vi "Untitled 13 (SubVI).vi"(4 "Порядок фильтра":i64, 5 "Array":dbl[](array[numeric]), 6 "Нижняя частота среза":dbl, 7 "Кол-во выборок":i32, 9 "Переменная floor(x/y)":i32, 10 "Кол-во копий":i32, 11 "Размер окна с паузами":i32) -> (3 "Filtered X":dbl[](array[numeric]))   [LabVIEW 2017]
uses:
  <vilib>/Analysis/3filter.llb/Bessel Filter (DBL).vi
  <vilib>/Analysis/NI_AALBase.lvlib
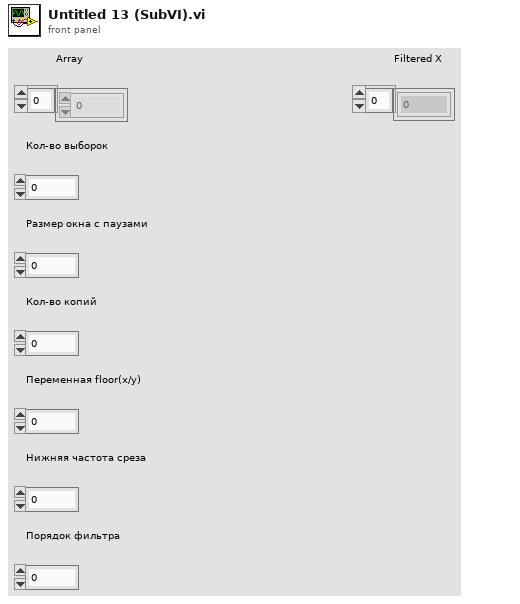
[diagram p1: front panel]
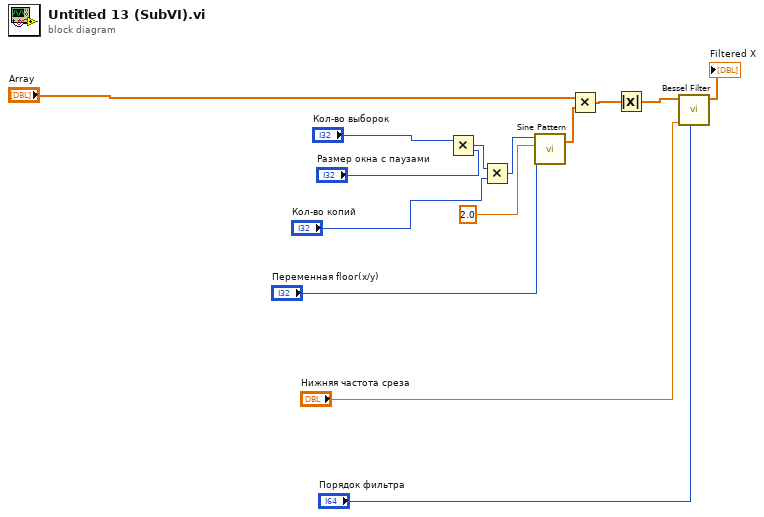
[diagram p0: block diagram]
diagram:
  n1 = Multiply(x="Кол-во выборок", y="Размер окна с паузами") -> (x*y=w12:i32)
  n2 = Multiply(x=w12, y="Кол-во копий") -> (x*y=w13:i32)
  n3 = call <vilib>:"Sine Pattern.vi"("cycles"="Переменная floor(x/y)", "amplitude"=2.0, "samples"=w13) -> ("Sinusoidal Pattern"=w7:dbl[])  [unwired: 1 in, 1 out]
  n4 = Multiply(x="Array", y=w7) -> (x*y=w3:dbl[])
  n5 = Absolute Value(x=w3) -> (abs(x)=w6:dbl[])
  n6 = call-poly <vilib>:"Bessel Filter.vi"("order"="Порядок фильтра", "low cutoff freq: fl"="Нижняя частота среза", "X"=w6) -> ("Filtered X"=→"Filtered X":dbl[])  [unwired: 5 in, 1 out]
